vi "Build HF Tasks.vi"(8 "error in":errorcluster, 11 "CRDS in":refnum<class "CRDS.lvclass">=refnum) -> (0 "error out":errorcluster, 3 "CRDS out":refnum<class "CRDS.lvclass">)   [LabVIEW 2012, in "CRDS.lvclass"]
doc: "Setup the high frequency signals. The YAG and Diode lasers are run off of the counters on the M-series board. The YAG is pulsed and the Diode is a square wave with a 50% duty cycle (or whatever the user defined DC). The YAG pulse will be initially triggered off of the falling edge of the diode laser. The YAG pulse will be routed internally through the InternalOutput terminal on the M-series board and connected to a counter on the S-series board using the PXI backplane. The pulse generated on the backplane will then gate the acquisition of the microphone and photodiode signals. Acquisition will occur only when the YAG signal is high."
uses:
  CRDS.lvclass
  <vilib>/DAQmx/create/channels.llb/DAQmx Create Channel (CO-Pulse Generation-Frequency).vi
  <vilib>/DAQmx/configure/timing.llb/DAQmx Timing (Implicit).vi
  <vilib>/DAQmx/configure/trigger.llb/DAQmx Start Trigger (Digital Edge).vi
  <resource>/objmgr/daqmx.rc
  Controls/Counter Descr.ctl
  Controls/Configuration/Counter Ctl.ctl
  Controls/Configuration/Cell Description.ctl
  <vilib>/DAQmx/configure/timing.llb/DAQmx Timing (Sample Clock).vi
  <vilib>/DAQmx/create/channels.llb/DAQmx Create Channel (AI-Voltage-Basic).vi
  PAS_CRDS new/CRDS/Controls/chDescr.ctl
  PAS_CRDS new/CRDS/Controls/las_lambda.ctl
  Cell Class/CRDS Cell.lvclass
  <vilib>/Utility/config.llb/NI_LVConfig.lvlib
  <vilib>/Utility/config.llb/Read Key (Boolean).vi
  PAS_CRDS new/CRDS/Controls/LaserAICluster.ctl
  PAS_CRDS new/CRDS/Controls/HF_AI Cfg.ctl
  <vilib>/Utility/config.llb/Read Key (Double).vi
  Instruments/cPAS/Interface/Controls/expFitMethod.ctl
  <vilib>/Utility/config.llb/Config Data RefNum.ctl
  Cell/Get Tau Method.ctl
  Base CRDS Lib.lvlib
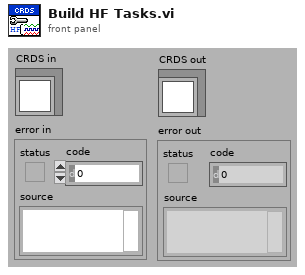
[diagram p1: front panel]
types:
  T1 = typedef "NI_LVConfig.lvlib/Config Data RefNum.ctl" = refnum<k1>
  T2 = typedef "LaserAICluster.ctl" = T3[]
  T3 = typedef "HF_AI Cfg.ctl" = cluster{"Channel":tag, "chDescr":T4, "Laser":T5, "Active":bool}
  T4 = typedef "chDescr.ctl" = enum16{"Ref", "Dry", "60%", "90%"}
  T5 = typedef "las_lambda.ctl" = enum16{"Red", "Blue", "Green"}
  T6 = typedef "Cell Description.ctl" = cluster{"fhkAI":dbl, "fai":dbl, "flas":dbl, "Analysis Method":T7, "Cavity Length":cluster{"Cell 1":dbl, "Cell 2":dbl, "Cell 3":dbl, "Cell 4":dbl, "Cell 5":dbl, "Cell 6":dbl, "Cell 7":dbl, "Cell 8":dbl}, "Wavelength":cluster{"Red":dbl, "Blue":dbl, "Green":dbl}}
  T7 = typedef "expFitMethod.ctl" = cluster{"Red":T8, "Blue":T8, "Green":T8}
  T8 = typedef "Base CRDS Lib.lvlib/Get Tau Method.ctl" = enum8{"DFT-1", "DFT-5", "LRS"}
  T9 = typedef "Counter Ctl.ctl" = cluster{"YAG":T10, "Diode":T10, "Gated":T10}
  T10 = typedef "Counter Descr.ctl" = cluster{"Counter":tag, "Duty Cycle":dbl}
  T11 = cluster{"Cell 1":dbl, "Cell 2":dbl, "Cell 3":dbl, "Cell 4":dbl, "Cell 5":dbl, "Cell 6":dbl, "Cell 7":dbl, "Cell 8":dbl}
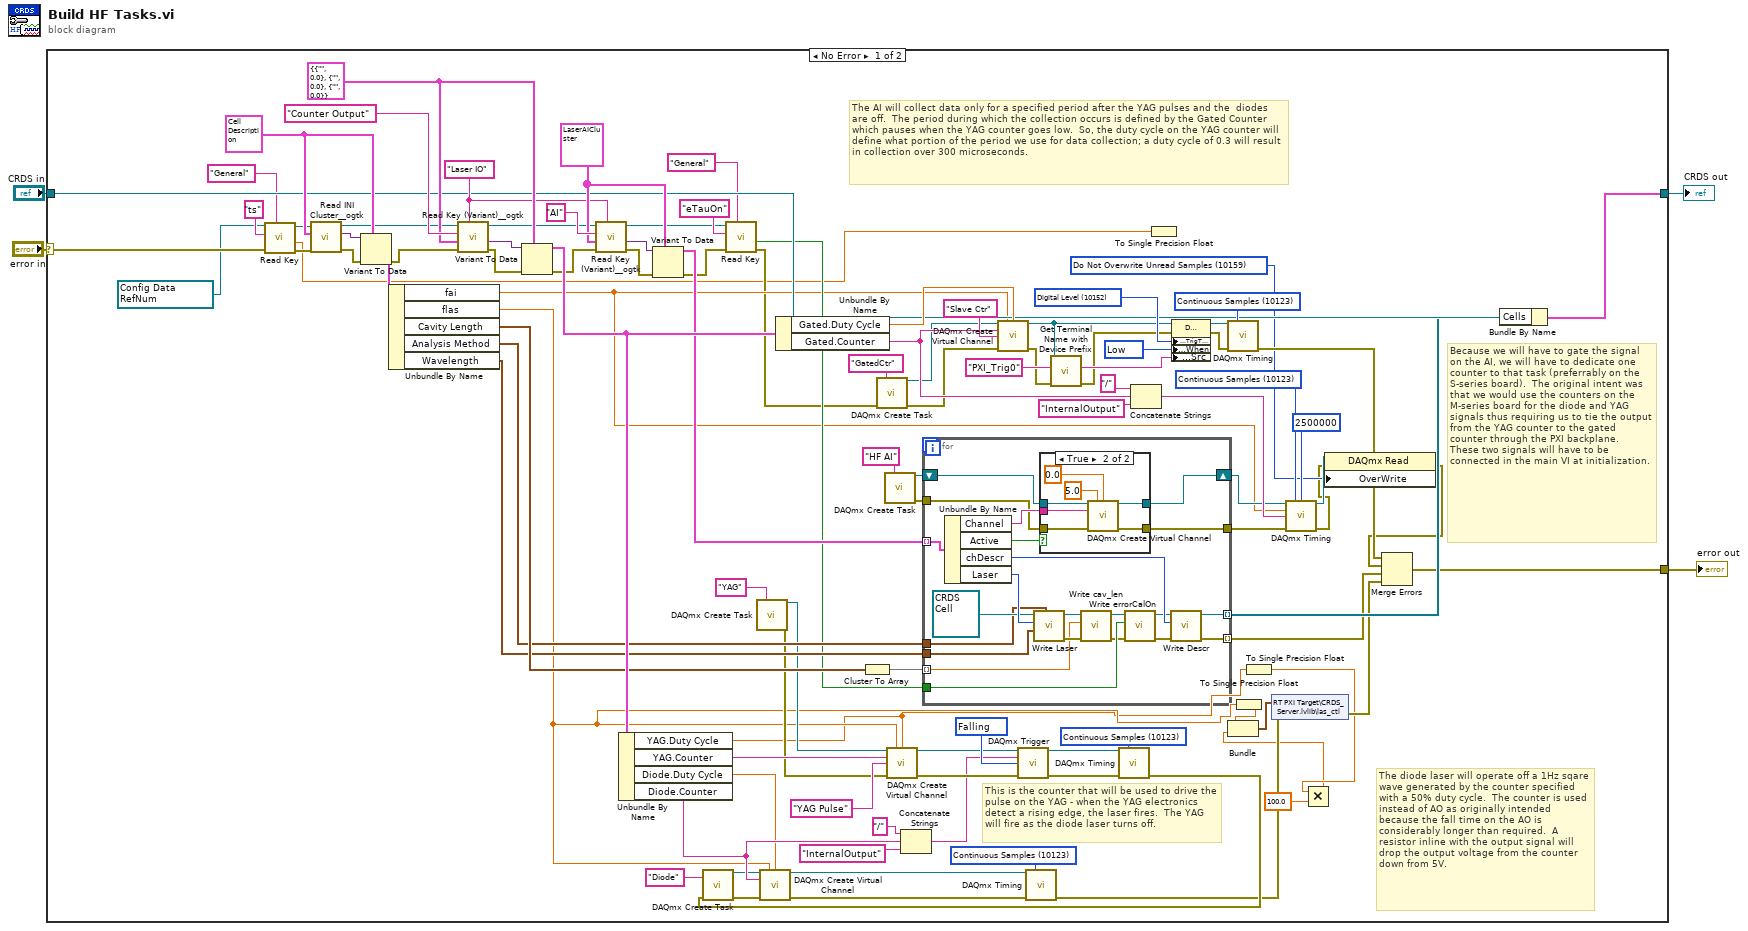
[diagram p0: block diagram]
diagram:
  n1 = case shown="No Error" "error in" {
    selector: "error in" -> [w37 w142]
    tunnel: [w40 w142] -> w3
    tunnel: [w65 w141] -> w1
    tunnel: "CRDS in" -> [w53 w141]
    frame No Error {
      w5 = T1 refnum items=["config data"] ("refnum")
      w8 = 10159 items=["Overwrite Unread Samples"=10252, "Do Not Overwrite Unread Samples"=10159] ("OverWrite")
      w61 = T2 [{"Channel"="", "chDescr"=enum."Ref", "Laser"=enum."Red", "Active"=FALSE}, {"Channel"="", "chDescr"=enum."Ref", "Laser"=enum."Red", "Active"=FALSE}, {"Channel"="", "chDescr"=enum."Ref", "Laser"=enum."Red", "Active"=FALSE}, {"Channel"="", "chDescr"=enum."Ref", "Laser"=enum."Red", "Active"=FALSE}, {"Channel"="", "chDescr"=enum."Ref", "Laser"=enum."Red", "Active"=FALSE}, {"Channel"="", "chDescr"=enum."Ref", "Laser"=enum."Red", "Active"=FALSE}, {"Channel"="", "chDescr"=enum."Ref", "Laser"=enum."Red", "Active"=FALSE}, {"Channel"="", "chDescr"=enum."Ref", "Laser"=enum."Red", "Active"=FALSE}] ("Laser AI")
      w73 = T6 {"fhkAI"=0.0, "fai"=0.0, "flas"=0.0, "Analysis Method"={"Red"=enum."DFT-1", "Blue"=enum."DFT-1", "Green"=enum."DFT-1"}, "Cavity Length"={"Cell 1"=0.0, "Cell 2"=0.0, "Cell 3"=0.0, "Cell 4"=0.0, "Cell 5"=0.0, "Cell 6"=0.0, "Cell 7"=0.0, "Cell 8"=0.0}, "Wavelength"={"Red"=0.0, "Blue"=0.0, "Green"=0.0}} ("Cell Setup")
      w74 = T9 {"YAG"={"Counter"="", "Duty Cycle"=0.0}, "Diode"={"Counter"="", "Duty Cycle"=0.0}, "Gated"={"Counter"="", "Duty Cycle"=0.0}} ("Counters")
      w59 = "Laser IO" ("section")
      w84 = 10123 items=["Finite Samples"=10178, "Continuous Samples"=10123, "Hardware Timed Single Point"=12522] ("sample mode")
      w91 = 10123 items=["Finite Samples"=10178, "Continuous Samples"=10123, "Hardware Timed Single Point"=12522] ("sample mode")
      w94 = 10214 items=["High"=10192, "Low"=10214] ("Pause.DigLvl.When")
      w95 = 10152 items=["Analog Level"=10101, "Analog Window"=10103, "Digital Level"=10152, "Digital Pattern"=10398, "None"=10230] ("Pause.TrigType")
      w97 = 10123 items=["Finite Samples"=10178, "Continuous Samples"=10123, "Hardware Timed Single Point"=12522] ("sample mode")
      w103 = 10171 items=["Rising"=10280, "Falling"=10171] ("edge")
      w106 = 10123 items=["Finite Samples"=10178, "Continuous Samples"=10123, "Hardware Timed Single Point"=12522] ("sample mode")
      # "Because we will have to gate the signal on the AI, we will have to dedicate one counter to that task (preferrably on the S-series board).  The original intent was that we would use the counters on the M-series board for the diode and YAG signals thus requiring us to tie the output from the YAG counter to the gated counter through the PXI backplane.   These two signals will have to be connected in the main VI at initialization."
      # "The AI will collect data only for a specified period after the YAG pulses and the  diodes are off.  The period during which the collection occurs is defined by the Gated Counter which pauses when the YAG counter goes low.  So, the duty cycle on the YAG counter will define what portion of the period we use for data collection; a duty cycle of 0.3 will result in collection over 300 microseconds."
      # "The diode laser will operate off a 1Hz sqare wave generated by the counter specified with a 50% duty cycle.  The counter is used instead of AO as originally intended because the fall time on the AO is considerably longer than required.  A resistor inline with the output signal will drop the output voltage from the counter down from 5V."
      # "This is the counter that will be used to drive the pulse on the YAG - when the YAG electronics detect a rising edge, the laser fires.  The YAG will fire as the diode laser turns off."
      n2 = call-poly <vilib>:"Read Key.vi"("section"="General", "error in (no error)"=w37, "key"="ts", "refnum"=w5) -> ("error out"=w38:errorcluster, "value"=w22:dbl, "refnum out"=w39:T1)  [unwired: 4 in, 1 out]
      n3 = call <userlib>:"Read INI Cluster__ogtk.vi"("error in (no error)"=w38, "INI Fomatted Cluster Type"=w73, "refnum"=w39) -> ("error out"=w70:errorcluster, "INI Fomatted Cluster"=w72:variant, "dup refnum"=w69:T1)  [unwired: 4 in, 2 out]
      n4 = Variant To Data(error in=w70, type=w73, Variant=w72) -> (data=w71:T6, error out=w68:errorcluster)
      n5 = Unbundle By Name(w71) -> ("fai"=w34:dbl, "flas"=w16:dbl, "Cavity Length"=w52:T11, "Analysis Method"=w50:T7, "Wavelength"=w49:cluster{"Red":dbl, "Blue":dbl, "Green":dbl})
      n6 = call <userlib>:"Read Key (Variant)__ogtk.vi"("section"=w59, "error in (no error)"=w68, "type"=w74, "key (optional)"="Counter Output", "refnum"=w69) -> ("error out"=w78:errorcluster, "key-value"=w76:variant, "refnum out"=w60:T1)  [unwired: 3 in, 1 out]
      n7 = Variant To Data(error in=w78, type=w74, Variant=w76) -> (data=w75:T9, error out=w20:errorcluster)
      n8 = call <userlib>:"Read Key (Variant)__ogtk.vi"("section"=w59, "error in (no error)"=w20, "type"=w61, "key (optional)"="AI", "refnum"=w60) -> ("error out"=w63:errorcluster, "key-value"=w64:variant, "refnum out"=w47:T1)  [unwired: 3 in, 1 out]
      n9 = Unbundle By Name(w75) -> ("YAG.Duty Cycle"=w14:dbl, "YAG.Counter"=w56:tag, "Diode.Duty Cycle"=w54:dbl, "Diode.Counter"=w55:tag)
      n10 = Variant To Data(error in=w63, type=w61, Variant=w64) -> (data=w58:T2, error out=w45:errorcluster)
      n11 = call-poly <vilib>:"Read Key.vi"("section"="General", "error in (no error)"=w45, "key"="eTauOn", "refnum"=w47) -> ("error out"=w31:errorcluster, "value"=w44:bool)  [unwired: 4 in, 2 out]
      n12 = call <vilib>:"DAQmx Create Task.vi"("new task name"="YAG") -> ("task out"=w29:refnum<k21>, "error out"=w28:errorcluster)  [unwired: 13 in]
      n13 = Unbundle By Name(w75) -> ("Gated.Duty Cycle"=w67:dbl, "Gated.Counter"=w66:tag)
      n14 = Cluster To Array(cluster=w52) -> (array=w51:dbl[])
      n15 = call <vilib>:"DAQmx Create Task.vi"("new task name"="GatedCtr", "error in"=w31) -> ("task out"=w32:refnum<k21>, "error out"=w30:errorcluster)  [unwired: 12 in]
      n16 = call <vilib>:"DAQmx Create Task.vi"("new task name"="HF AI") -> ("task out"=w109:refnum<k21>, "error out"=w107:errorcluster)  [unwired: 13 in]
      n17 = call-poly <vilib>:"DAQmx Create Virtual Channel.vi"("task in"=w29, "frequency"=w16, "duty cycle"=w14, "counter"=w56, "name to assign"="YAG Pulse", "error in"=w28) -> ("task out"=w102:refnum<k21>, "error out"=w99:errorcluster)  [unwired: 8 in]
      n18 = Concatenate Strings("/", w55, "InternalOutput" ("string")) -> (w98:string)
      n19 = for {
        tunnel: w58 -> [w131] mode=indexing
        shift-right: [w126] -> w85
        shift-left: w109 -> [w129]
        tunnel: w107 -> [w128]
        tunnel: [w127] -> w43
        tunnel: w51 -> [w120] mode=indexing
        tunnel: w50 -> [w119]
        tunnel: w49 -> [w118]
        tunnel: w44 -> [w117]
        tunnel: [w114] -> w42 mode=indexing
        tunnel: [w113] -> w21 mode=indexing
        n20 = Unbundle By Name(w131) -> ("Channel"=w130:tag, "Active"=w125:bool, "chDescr"=w112:T4, "Laser"=w124:T5)
        n21 = call "Write Laser.vi"("analisysMeth"=w119, "Wavelength"=w118, "Laser"=w124, "CRDS Cell in"=refnum<class "CRDS Cell.lvclass"> refnum) -> ("error out"=w121:errorcluster, "CRDS Cell out"=w122:refnum<class "CRDS Cell.lvclass">)  [unwired: 6 in]
        n22 = case shown="True" w125 {
          tunnel: w130 -> [_ w140]
          tunnel: w129 -> [w133 w139]
          tunnel: w128 -> [w132 w138]
          tunnel: [w132 w137] -> w127
          tunnel: [w133 w136] -> w126
          frame False {
          }
          frame True {
            n23 = call-poly <vilib>:"DAQmx Create Virtual Channel.vi"("task in"=w139, "maximum value"=5.0, "minimum value"=0.0, "physical channels"=w140, "error in"=w138) -> ("task out"=w136:refnum<k21>, "error out"=w137:errorcluster)  [unwired: 9 in]
          }
        }
        n24 = call "Write cav_len.vi"("error in (no error)"=w121, "cav_len"=w120, "CRDS Cell in"=w122) -> ("error out"=w115:errorcluster, "CRDS Cell out"=w116:refnum<class "CRDS Cell.lvclass">)  [unwired: 7 in]
        n25 = call "Write errorCalOn.vi"("error in (no error)"=w115, "errorCalOn"=w117, "CRDS Cell in"=w116) -> ("error out"=w110:errorcluster, "CRDS Cell out"=w111:refnum<class "CRDS Cell.lvclass">)  [unwired: 7 in]
        n26 = call "Write Descr.vi"("error in (no error)"=w110, "Descr"=w112, "CRDS Cell in"=w111) -> ("error out"=w113:errorcluster, "CRDS Cell out"=w114:refnum<class "CRDS Cell.lvclass">)  [unwired: 7 in]
      }
      n27 = call-poly <vilib>:"DAQmx Create Virtual Channel.vi"("task in"=w32, "frequency"=w34, "duty cycle"=w67, "counter"=w66, "name to assign"="Slave Ctr", "error in"=w30) -> ("task out"=w81:refnum<k21>, "error out"=w80:errorcluster)  [unwired: 3 in, 5 out]
      n28 = call-poly <vilib>:"DAQmx Trigger.vi"("task/channels in"=w102, "source"=w98, "edge"=w103, "error in"=w99) -> ("task out"=w83:refnum<k21>, "error out"=w82:errorcluster)  [unwired: 10 in]
      n29 = call "Get Terminal Name with Device Prefix.vi"("error in (no error)"=w80, "Local Terminal Name"="PXI_Trig0", "task/channels in"=w81) -> ("error out"=w79:errorcluster, "Terminal Name with Device Prefix"=w89:tag)  [unwired: 6 in, 1 out]
      n30 = call-poly <vilib>:"DAQmx Timing.vi"("task/channels in"=w83, "sample mode"=w84, "error in"=w82) -> ("error out"=w23:errorcluster)  [unwired: 11 in, 1 out]
      n31 = call <vilib>:"DAQmx Create Task.vi"("new task name"="Diode", "error in"=w23) -> ("task out"=w26:refnum<k21>, "error out"=w25:errorcluster)  [unwired: 12 in]
      n32 = call-poly <vilib>:"DAQmx Create Virtual Channel.vi"("task in"=w26, "frequency"=w16, "duty cycle"=w54, "counter"=w55, "error in"=w25) -> ("task out"=w104:refnum<k21>, "error out"=w105:errorcluster)  [unwired: 9 in]
      n33 = call-poly <vilib>:"DAQmx Timing.vi"("task/channels in"=w104, "sample mode"=w106, "error in"=w105) -> ("error out"=w18:errorcluster)  [unwired: 11 in, 1 out]
      n34 = Concatenate Strings("/", w66, "InternalOutput" ("string")) -> (w86:string)
      n35 = To Single Precision Float(number=w22) -> ()  [unwired: 1 out]
      n36 = property class="DAQmx Trigger"(reference=w81, error in=w79, "Pause.TrigType"=w95, "Pause.DigLvl.When"=w94, "Pause.DigLvl.Src"=w89) -> (reference out=w93:refnum<k21>, error out=w92:errorcluster)
      n37 = call-poly <vilib>:"DAQmx Timing.vi"("task/channels in"=w93, "sample mode"=w91, "error in"=w92) -> ("error out"=w41:errorcluster)  [unwired: 1 in, 11 out]
      n38 = To Single Precision Float(number=w16) -> (single precision float=w15:sgl)
      n39 = To Single Precision Float(number=w14) -> (single precision float=w12:sgl)
      n40 = call-poly <vilib>:"DAQmx Timing.vi"("task/channels in"=w85, "sample mode"=w97, "samples per channel"=2500000, "rate"=w34, "source"=w86, "error in"=w43) -> ("task out"=w9:refnum<k21>, "error out"=w7:errorcluster)  [unwired: 1 in, 7 out]
      n41 = Multiply(x=w12, y=sgl 100.0) -> (x*y=w11:sgl)
      n42 = Bundle(w15, w11) -> (w19:cluster{sgl, sgl})  [unwired: 1 in]
      n43 = shared-variable "RT PXI Target\\CRDS_Server.lvlib\\las_ctl"(w19, error in=w18) -> (error out=w17:errorcluster)
      n44 = property class="DAQmx Read"(reference=w9, error in=w7, "OverWrite"=w8) -> (error out=w6:errorcluster)  [unwired: 1 out]
      n45 = Merge Errors(w41, w6, w21, w17) -> (w40:errorcluster)
      n46 = Bundle By Name(cluster=w53, "Cells"=w42) -> (w65:cluster{})
    }
    frame Error {
    }
  }
  "error out" <- w3
  "CRDS out" <- w1
